vi "run.vi"(8 "error in (no error)":errorcluster, 10 "Input":string, 11 "Packet in":refnum<class "RPCFunction.lvclass">) -> (0 "error out":errorcluster, 2 "Output":string, 3 "Packet out":refnum<class "RPCFunction.lvclass">)   [LabVIEW 2011, in "mbed_LVLibrary.lvlib" / "RPCFunction.lvclass"]
uses:
  RPCFunction.lvclass
  RPCFunction.lvclass/RPCFunction.ctl
  Transport Mechanisms/mbed/mbed.lvclass
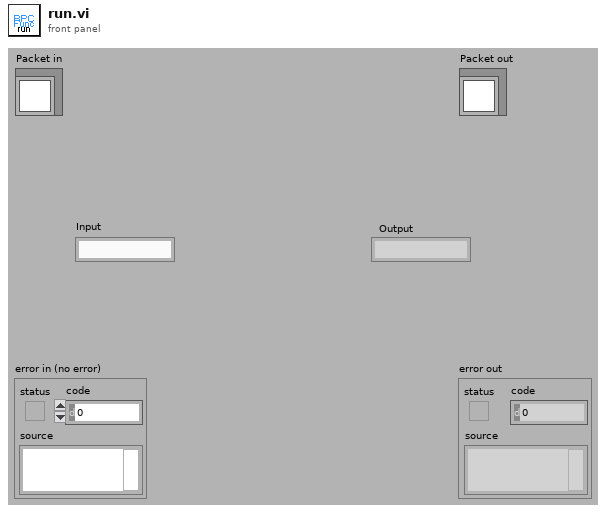
[diagram p1: front panel]
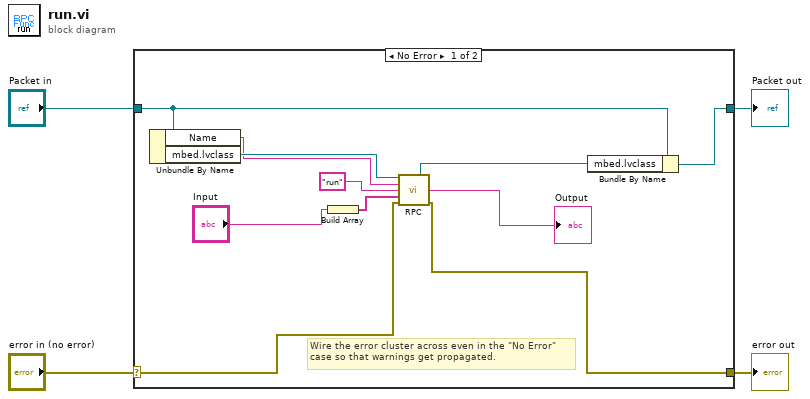
[diagram p0: block diagram]
diagram:
  n1 = case shown="No Error" "error in (no error)" {
    selector: "error in (no error)" -> [w7 w17]
    tunnel: [w6 w17] -> w3
    tunnel: [w14 w16] -> w1
    tunnel: "Packet in" -> [w15 w16]
    frame No Error {
      # "Wire the error cluster across even in the \"No Error\"\ncase so that warnings get propagated."
      n2 = Unbundle By Name(w15) -> ("Name"=w12:string, "mbed.lvclass"=w13:refnum<class "mbed.lvclass">)
      n3 = Build Array("Input") -> (w9:string[])
      n4 = call-dynamic "RPC.vi"("mbed in"=w13, "Name"=w12, "method"="run", "Args"=w9, "error in (no error)"=w7) -> ("mbed out"=w11:refnum<class "mbed.lvclass">, "RPC Result"=→"Output":string, "error out"=w6:errorcluster)  [unwired: 8 in]
      n5 = Bundle By Name(cluster=w15, "mbed.lvclass"=w11) -> (w14:refnum<class "RPCFunction.lvclass">)
    }
    frame Error {
    }
  }
  "error out" <- w3
  "Packet out" <- w1
